vi "Test Process Error Handler Process Context When Set.vi"(8 "error in (no error)":errorcluster, 11 "Process Dev Test in":refnum<class "Process Dev Test.lvclass">) -> (0 "error out":errorcluster, 3 "Process Dev Test out":refnum<class "Process Dev Test.lvclass">)   [LabVIEW 2020, in "Process Dev Test.lvclass"]
uses:
  Process Dev Test.lvclass
  C:/Program Files (x86)/National Instruments/LabVIEW 2020/vi.lib/Astemes/LUnit/Test Case.lvclass
  source/Framework/Process/Process.lvclass
  source/Framework Test Suite/Mock Process/Mock Process.lvclass
  C:/Git/triarc-framework/source/Framework/Error Handler Interface/Error Handler Interface.lvclass
  source/Framework/Process/Process.lvclass/Process.ctl
  <vilib>/Astemes/LUnit/Test Case.lvclass/Test Case.ctl
  2667621f-421a-4321-bcf2-66b0418d2e0c.vi
  source/Framework/Process/Protected/Messaging/Send Message.vi
  source/Framework/Process/Public/Lifecycle/Get Lifecycle State.vi
  source/Framework/Process/Protected/SubVIs/Set Context.vi
  <vilib>/Utility/error.llb/Clear Errors.vi
  <vilib>/Astemes/LUnit/Palette/Pass.vi
  <vilib>/Astemes/LUnit/Palette/Fail.vi
  <vilib>/Astemes/LUnit/Compare Variants.vi
  <vilib>/Astemes/LUnit/Describe Comparison.vi
  <vilib>/Astemes/LUnit/Set Assertion Type.vi
  source/Framework/Process/Private/SubVIs/Handle Debug Data.vi
  source/Framework/Process/Public/Lifecycle/Leave Process Loop.vi
  <vilib>/Astemes/LUnit/Add test result.vi
  <vilib>/Astemes/LUnit/Variant to string.vi
  <vilib>/Utility/High Resolution Relative Seconds.vi
  <vilib>/Astemes/LUnit/LUnit Record Assertion Result.vi
  <vilib>/Astemes/LUnit/LUnit Aggregate Assertion Results.vi
  <vilib>/Astemes/LUnit/Method Result/LUnit Merge Status.vi
  <vilib>/Astemes/LUnit/LUnit Concatenate result strings.vi
  <vilib>/Utility/error.llb/Error Cluster From Error Code.vi
  <vilib>/Utility/Data Type/Get Type Information.vi
  <vilib>/Utility/LVClass/Get LV Class Name.vi
panel:
  out "Qualified Name":string
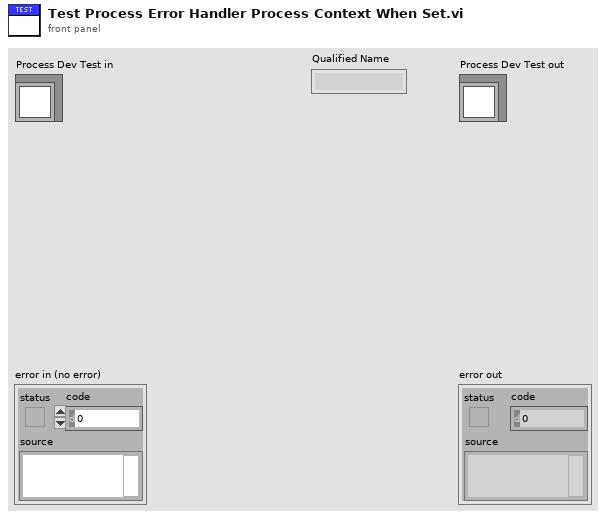
[diagram p1: front panel]
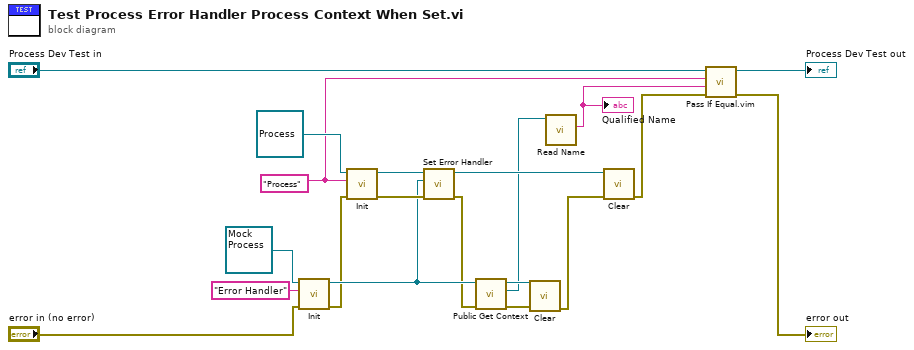
[diagram p0: block diagram]
diagram:
  w1 = "Process" ("Name")
  n1 = call-dynamic "Init.vi"("error in (no error)"="error in (no error)", "Name"="Error Handler", "Mock Process In"=refnum<class "Mock Process.lvclass"> refnum ("Mock Process.lvclass")) -> ("error out"=w9:errorcluster, "Mock Process Out"=w13:refnum<class "Mock Process.lvclass">)  [unwired: 7 in]
  n2 = call-dynamic "Init.vi"("error in (no error)"=w9, "Name"=w1, "Process In"=refnum<class "Process.lvclass"> refnum ("Process.lvclass")) -> ("error out"=w16:errorcluster, "Process Out"=w17:refnum<class "Process.lvclass">)  [unwired: 7 in]
  n3 = call "Set Error Handler.vi"("error in (no error)"=w16, "Error Handler"=w13, "Process In"=w17) -> ("error out"=w12:errorcluster, "Process Out"=w15:refnum<class "Process.lvclass">)  [unwired: 7 in]
  n4 = call "Public Get Context.vi"("error in (no error)"=w12, "Mock Process in"=w13) -> ("error out"=w14:errorcluster, "Context"=w3:refnum<class "Process.lvclass">, "Mock Process out"=w10:refnum<class "Mock Process.lvclass">)  [unwired: 7 in]
  n5 = call-dynamic "Clear.vi"("error in (no error)"=w14, "Mock Process In"=w10) -> ("error out"=w11:errorcluster)  [unwired: 9 in]
  n6 = call "Read Name.vi"("Process In"=w3) -> ("Qualified Name"=w2:string)  [unwired: 7 in, 3 out]
  "Qualified Name" <- w2
  n7 = call-dynamic "Clear.vi"("error in (no error)"=w11, "Process In"=w15) -> ("error out"=w7:errorcluster)  [unwired: 9 in]
  n8 = call "Pass If Equal.vim"("error in (no error)"=w7, "Actual"=w2, "Expected"=w1, "LUnit Test Case In"="Process Dev Test in") -> ("error out"=→"error out":errorcluster, "LUnit Test Case Out"=→"Process Dev Test out":refnum<class "Process Dev Test.lvclass">)  [unwired: 6 in]
